vi "Read Initialization.vi"(8 "error in (no error)":errorcluster, 11 "CCD in":refnum<class "CCD.lvclass">) -> (0 "error out":errorcluster, 2 "Initialization":bool, 3 "CCD out":refnum<class "CCD.lvclass">)   [LabVIEW 2018, in "CCD.lvclass"]
uses:
  CCD.lvclass
  CCD.lvclass/CCD.ctl
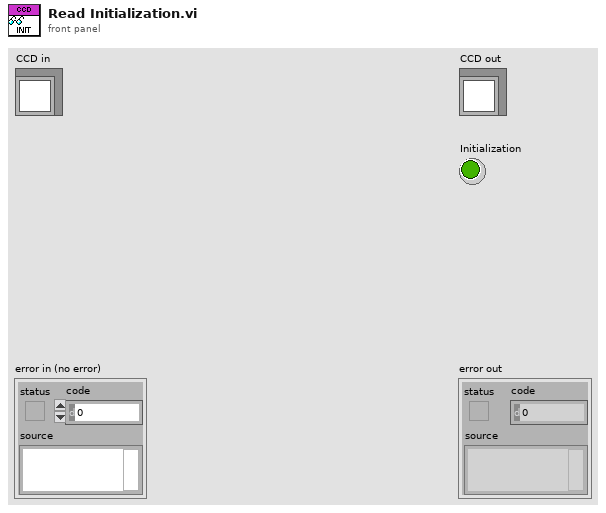
[diagram p1: front panel]
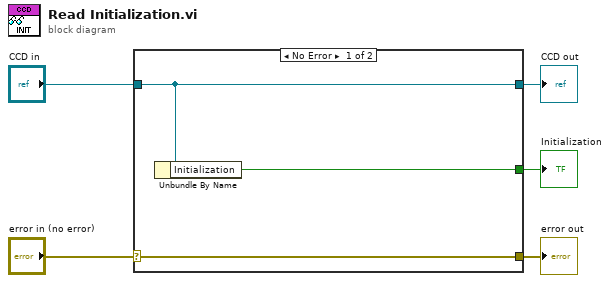
[diagram p0: block diagram]
diagram:
  n1 = case shown="No Error" "error in (no error)" {
    selector: "error in (no error)" -> [w8 w9]
    tunnel: [w8 w9] -> w4
    tunnel: [w7 w10] -> w2
    tunnel: "CCD in" -> [w7 w10]
    tunnel: [w6 _] -> w1
    frame No Error {
      n2 = Unbundle By Name(w7) -> ("Initialization"=w6:bool)
    }
    frame Error {
    }
  }
  "error out" <- w4
  "CCD out" <- w2
  "Initialization" <- w1
